vi "Test Pass on Expected Element in Map.vi"(8 "error in (no error)":errorcluster, 11 "LUnit Test Case V2 Test Double In":refnum<class "Test Case Test Double.lvclass">) -> (0 "error out":errorcluster, 3 "LUnit Test Case V2 Test Double Out":refnum<class "Test Case Test Double.lvclass">)   [LabVIEW 2020, in "Test Case Test Double.lvclass"]
uses:
  Test Case Test Double.lvclass
  C:/git/astemes-lunit/source/LUnit Test Case.lvclass
  source/LUnit Test Case.lvclass/LUnit Test Case.ctl
  c6274006-89c2-48a4-8874-7a48b9f3ce57.vi
  source/Core/LUnit Test Case/Assertions/Pass If.vi
  source/Core/LUnit Test Case/Private/Append Fail Result.vi
  source/Core/LUnit Test Case/Private/Append Pass Result.vi
  source/Core/LUnit Test Case/Private/Run In UI.vi
  <vilib>/Utility/error.llb/Clear Errors.vi
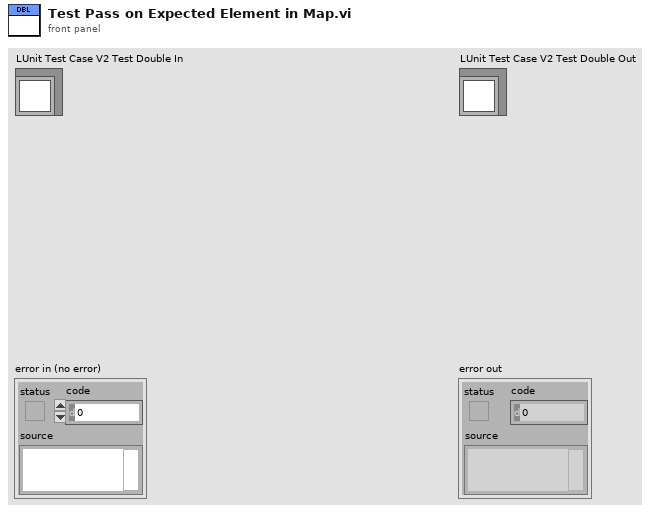
[diagram p1: front panel]
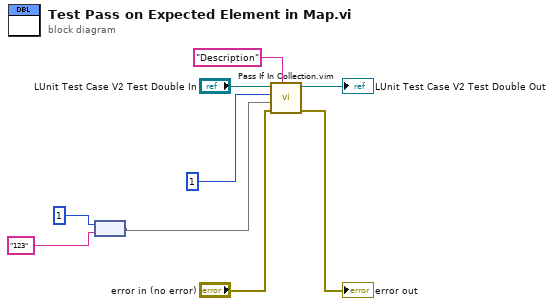
[diagram p0: block diagram]
diagram:
  n1 = node(1, "123") -> (w1:map{i32, string})
  n2 = call "Pass If In Collection.vim"("Description"="Description", "error in (no error)"="error in (no error)", "Collection"=w1, "Expected Element"=1, "LUnit Test Case In"="LUnit Test Case V2 Test Double In") -> ("error out"=→"error out":errorcluster, "LUnit Test Case Out"=→"LUnit Test Case V2 Test Double Out":refnum<class "Test Case Test Double.lvclass">)  [unwired: 5 in]
